vi "Delay_time.vi"() -> ()   [LabVIEW 2020]
doc: "Liczy czas kiedy pojazd jest poza pozycj¹."
panel:
  in  "Numeric":dbl
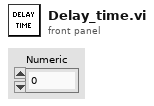
[diagram p1: front panel]
diagram:
